vi "PulseGen_USB_VISA_Bulk.vi"(8 "error in":errorcluster, 9 "Command Index":T1(ring), 10 "Numeric Input (Optional)":sgl, 11 "Resource Name":string) -> (0 "error out":errorcluster, 2 "read buffer":string, 3 "Resource Name 2":string)   [LabVIEW 2015]
doc: "Commands\n 0 - set units (0-inHg, 1-mmHg, 2-torr, 3-mbar)\n 1 - set vacuum zero\n 2 - reserved\n 3 - reserved\n 4 - reserved\n 5 - set vacuum calibration\n 6 - reserved\n 7 - start bootloader\n 8 - get firmware version\n 9 - get vacuum reading\n 10 - start/stop vacuum control (0-stop, 1-start)\n 11 - set vacuum setpoint\n 12 - set calibration zero offset (prevent negative zero value from DWIN)\n 13 - set pump speed 0-100 \n 14 - set vacuum valve PWM 0-1000\n 15 - set bleed valve PWM 0-1000"
panel:
  out "concatenated string":string
  out "value":sgl
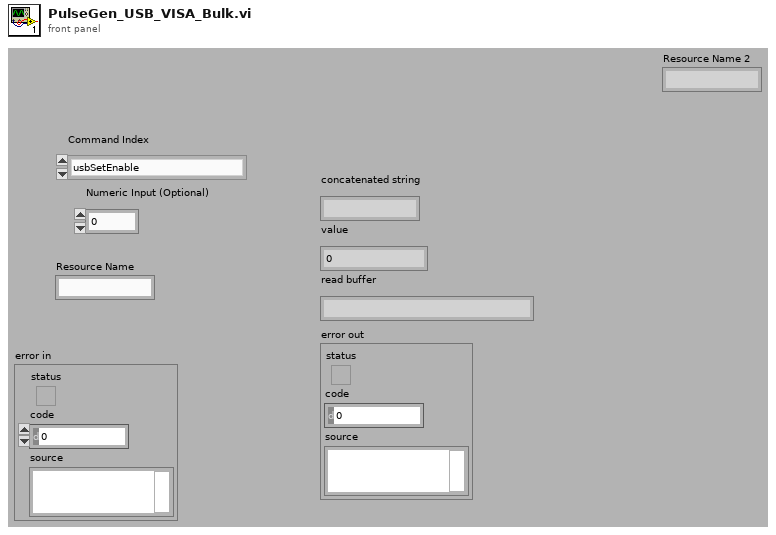
[diagram p1: front panel]
types:
  T1 = enum16{"usbSetEnable", "usbSetDirection", "usbSetCounts", "usbSetClock", "usbStartMotion"}
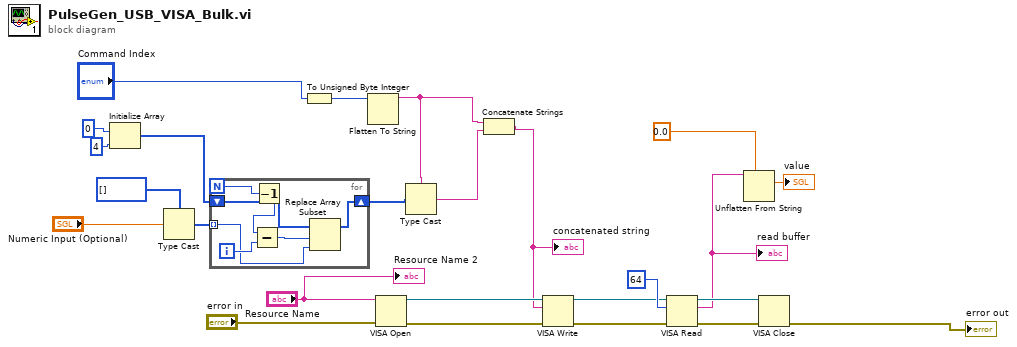
[diagram p0: block diagram]
diagram:
  n1 = Initialize Array(u8 0, 4 ("dimension size")) -> (w10:u8[])
  n2 = Type Cast(type=u8[] [], x="Numeric Input (Optional)") -> (*(type *) &x=w14:u8[])
  n3 = for {
    N -> [w28]
    tunnel: w14 -> [w31] mode=indexing
    shift-right: [w29] -> w9
    shift-left: w10 -> [w30]
    i -> [w32]
    n4 = Decrement(x=w28) -> (x-1=w27:i32)
    n5 = Subtract(x=w27, y=w32) -> (x-y=w26:i32)
    n6 = Replace Array Subset(array=w30, new element=w31, index=w26) -> (w29:u8[])
  }
  n7 = To Unsigned Byte Integer(number="Command Index") -> (unsigned 8bit integer=w4:u8)
  n8 = Flatten To String(anything=w4) -> (data string=w8:string)  [unwired: 3 in, 2 out]
  n9 = VISA Open(error in (no error)="error in", VISA resource name="Resource Name") -> (VISA resource name=w24:refnum<visa-resource-name>, error out=w25:errorcluster)  [unwired: 3 out]
  n10 = Type Cast(type=w8, x=w9) -> (*(type *) &x=w6:string)
  n11 = Concatenate Strings(w8, w6) -> (w7:string)
  "concatenated string" <- w7
  n12 = VISA Write(VISA resource name=w24, write buffer=w7, error in (no error)=w25) -> (VISA resource name out=w21:refnum<visa-resource-name>, error out=w22:errorcluster)  [unwired: 1 out]
  n13 = VISA Read(VISA resource name=w21, byte count=u32 64 ("Bytes To Read"), error in (no error)=w22) -> (VISA resource name out=w19:refnum<visa-resource-name>, read buffer=w18:string, error out=w20:errorcluster)  [unwired: 1 out]
  "read buffer" <- w18
  n14 = Unflatten From String(type=sgl 0.0, binary string=w18) -> (value=→"value":sgl)  [unwired: 3 in, 2 out]
  n15 = VISA Close(VISA resource name=w19, error in (no error)=w20) -> (error out=→"error out":errorcluster)
  "Resource Name 2" <- "Resource Name"
